vi "Create Command.vi"(8 "error in (no error)":errorcluster, 11 "message refnum in":T1=18446744073709551615 format="%.0x") -> (0 "error out":errorcluster, 2 "response refnum":T1=18446744073709551615 format="%.0x", 3 "message refnum out":T1=18446744073709551615 format="%.0x")   [LabVIEW 2020, in "Scripting API.lvlib"]
uses:
  Scripting API.lvlib
  <vilib>/NI VeriStand/Custom Device API/Custom Device Item Ref.ctl
  <vilib>/NI VeriStand/Custom Device API/Custom Device API.lvlib
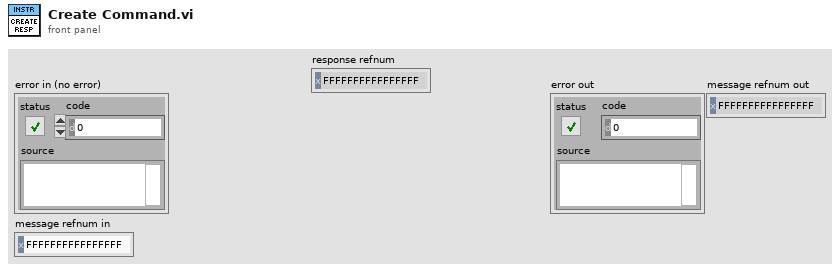
[diagram p1: front panel]
types:
  T1 = typedef "Custom Device API.lvlib/Custom Device Item Ref.ctl" = u64
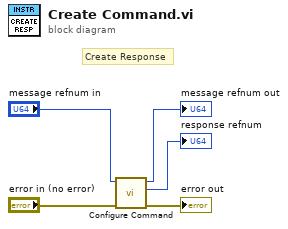
[diagram p0: block diagram]
diagram:
  # "Create Response"
  n1 = call "Configure Command.vi"("Error In"="error in (no error)", "C Refnum In"="message refnum in") -> ("Error Out"=→"error out":errorcluster, "Command Refnum"=→"response refnum":T1, "Message Refnum Out"=→"message refnum out":T1)  [unwired: 7 in]
